vi "Get Queue Attributes.vi"(8 "error in (no error)":errorcluster, 10 "Attributes":T2[](array[typedef])=[enum."All"], 11 "SQS in":refnum<class "SQS.lvclass">) -> (0 "error out":errorcluster, 2 "Attribute Results":T1[](array[typedef]), 3 "SQS out":refnum<class "SQS.lvclass">)   [LabVIEW 2015, in "NI_SQS.lvlib" / "SQS.lvclass"]
uses:
  SQS.lvclass
  Queue Attribute.ctl
  Attribute Value Pair.ctl
  Core/Name Value Pair.ctl
  Core/Request Options.ctl
  SQS.lvclass/SQS.ctl
  Read Account Number.vi
  Read Name.vi
  Core/NI_AWS Core.lvlib
  NI_SQS.lvlib
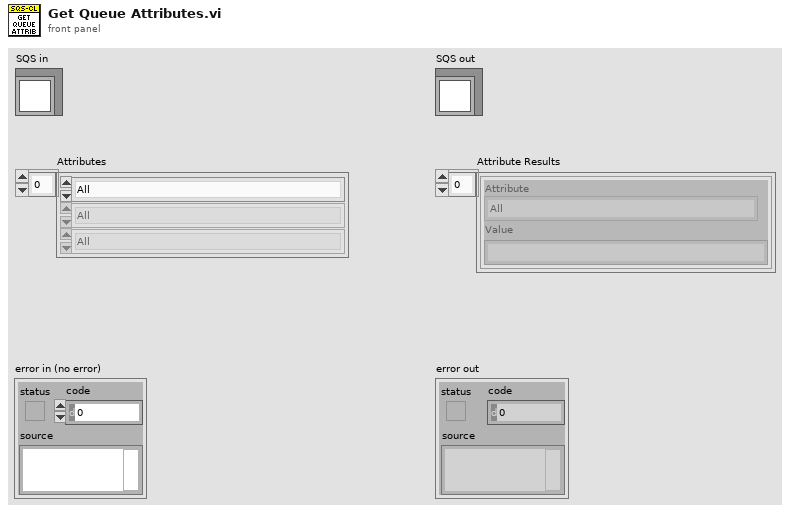
[diagram p1: front panel]
types:
  T1 = typedef "NI_SQS.lvlib/Attribute Value Pair.ctl" = cluster{"Attribute":T2, "Value":string}
  T2 = typedef "NI_SQS.lvlib/Queue Attribute.ctl" = enum16{"All", "Policy", "VisibilityTimeout", "MaximumMessageSize", "MessageRetentionPeriod", "ApproximateNumberOfMessages", "ApproximateNumberOfMessagesNotVisible", "CreatedTimestamp", "LastModifiedTimestamp", "QueueArn", "ApproximateNumberOfMessagesDelayed", "DelaySeconds", "ReceiveMessageWaitTimeSeconds", "RedrivePolicy", "FifoQueue", "ContentBasedDeduplication"}
  T3 = typedef "NI_AWS Core.lvlib/Request Options.ctl" = cluster{"request headers":T4[], "request parameters":T4[], "request body":string}
  T4 = typedef "NI_AWS Core.lvlib/Name Value Pair.ctl" = cluster{"name":string, "value":string}
  T5 = typedef "NI_AWS Core.lvlib/Response.ctl" = cluster{"Headers":string, "Body":string}
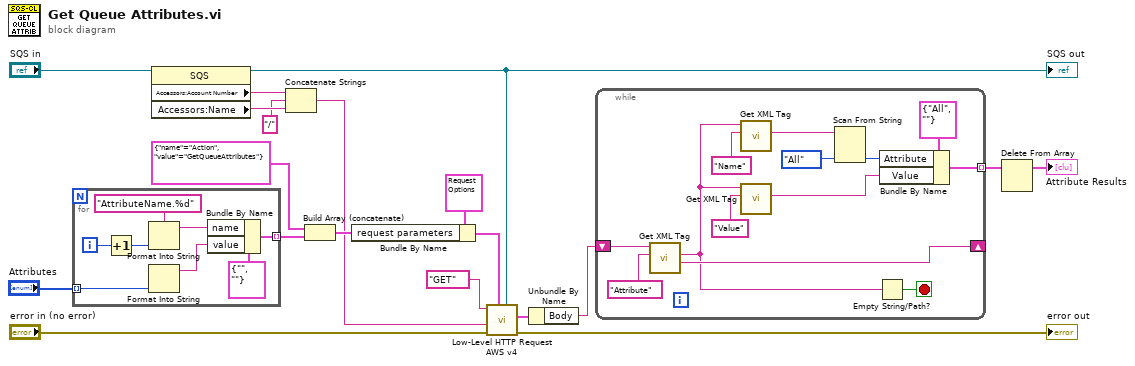
[diagram p0: block diagram]
diagram:
  n1 = for {
    tunnel: "Attributes" -> [w21] mode=indexing
    tunnel: [w22] -> w6 mode=indexing
    i -> [w27]
    n2 = Increment(x=w27) -> (x+1=w26:i32)
    n3 = Format Into String(format string="AttributeName.%d", w26) -> (resulting string=w23:string)  [unwired: 2 in, 1 out]
    n4 = Format Into String(w21) -> (resulting string=w20:string)  [unwired: 3 in, 1 out]
    n5 = Bundle By Name(cluster=T4 {"name"="", "value"=""} ("element"), "name"=w23, "value"=w20) -> (w22:T4)
  }
  n6 = property class="SQS"(reference="SQS in") -> (reference out=w5:refnum<class "SQS.lvclass">, "Accessors:Account Number"=w4:string, "Accessors:Name"=w3:string)  [unwired: 1 in, 1 out]
  "SQS out" <- w5
  n7 = Concatenate Strings(w4, "/", w3) -> (w1:string)
  n8 = Build Array (concatenate)(T4 {"name"="Action", "value"="GetQueueAttributes"} ("Cluster"), w6) -> (w7:T4[])
  n9 = Bundle By Name(cluster=T3 {"request headers"=[], "request parameters"=[{"name"="Action", "value"="ListQueues"}], "request body"=""} ("Request Options"), "request parameters"=w7) -> (w8:T3)
  n10 = call "Low-Level HTTP Request AWS v4.vi"("AWS Core"=w5, "Request Options"=w8, "error in (no error)"="error in (no error)", "URL Suffix"=w1, "HTTP-Verb"="GET") -> ("error out"=→"error out":errorcluster, "Response"=w15:T5)  [unwired: 4 in, 1 out]
  n11 = Unbundle By Name(w15) -> ("Body"=w14:string)
  n12 = while {
    shift-right: [w39] -> _
    shift-left: w14 -> [w40]
    tunnel: [w32] -> w13 mode=indexing
    stop <- w38 stop-if-true
    n13 = call "Get XML Tag.vi"("Tag name"="Attribute", "XML String in"=w40) -> ("Remaining string"=w39:string, "Tag value"=w34:string)  [unwired: 5 in, 3 out]
    n14 = call "Get XML Tag.vi"("Tag name"="Name", "XML String in"=w34) -> ("Tag value"=w30:string)  [unwired: 5 in, 4 out]
    n15 = call "Get XML Tag.vi"("Tag name"="Value", "XML String in"=w34) -> ("Tag value"=w31:string)  [unwired: 5 in, 4 out]
    n16 = Scan From String(input string=w30, default 1=Queue_Attribute."All" ("Attribute")) -> (output 1=w29:T2)  [unwired: 3 in, 3 out]
    n17 = Empty String/Path?(string/path=w34) -> (empty?=w38:bool)
    n18 = Bundle By Name(cluster=T1 {"Attribute"=enum."All", "Value"=""} ("Attribute Value Pair"), "Attribute"=w29, "Value"=w31) -> (w32:T1)
  }
  n19 = Delete From Array(array=w13) -> (array with subset deleted=→"Attribute Results":T1[])  [unwired: 2 in, 1 out]
